vi "JoystickLevel.vi"() -> ()   [LabVIEW 2016]
panel:
  in  "stop":bool
  out "Output":dbl
  in  "MidPower":dbl
  in  "StopThreshold":dbl
  in  "StartThreshold":dbl
  in  "Joystick":dbl(slide) min=-1.0 step=0.01 scale=-1.0..1.0
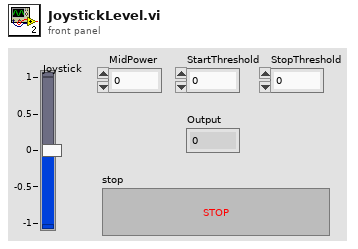
[diagram p1: front panel]
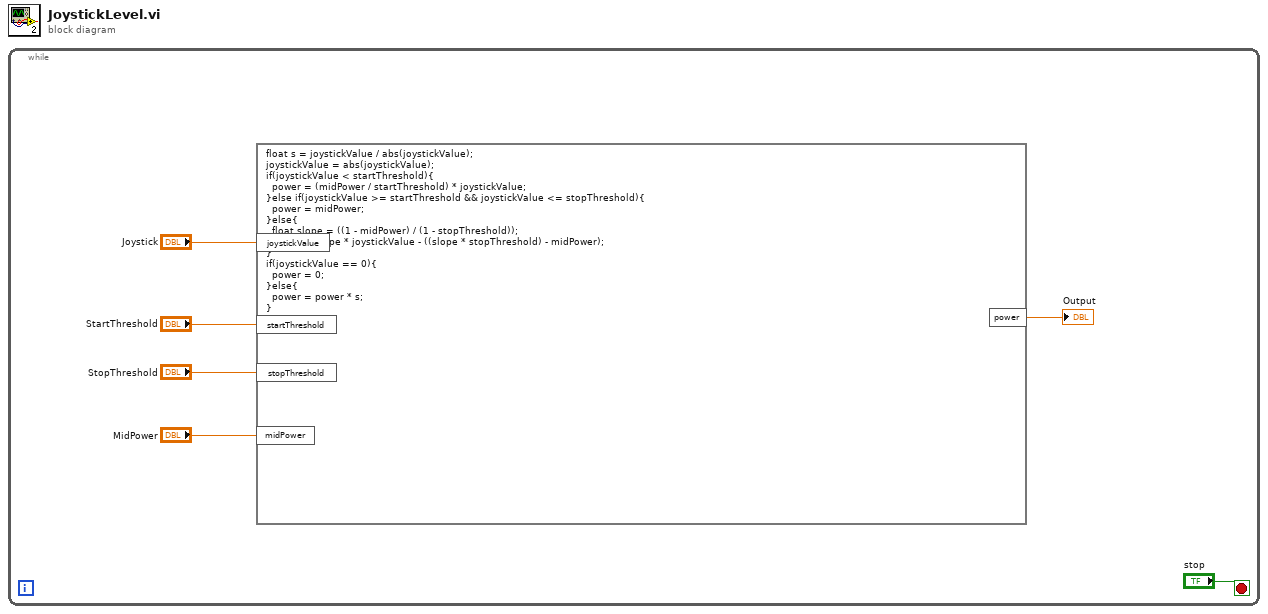
[diagram p0: block diagram]
diagram:
  n1 = while {
    stop <- "stop" stop-if-true
    n2 = formula code="float s = joystickValue / abs(joystickValue);\njoystickValue = abs(joystickValue);\nif(joystickValue < startThreshold){\n  power = (midPower / startThreshold) * joystickValue;\n}else if(joystickValue >= startThreshold && joystickValue <= stopThreshold){\n  power = midPower;\n}else{\n  float slope = ((1 - midPower) / (1 - stopThreshold));\n  power = slope * joystickValue - ((slope * stopThreshold) - midPower);\n}\nif(joystickValue == 0){\n  power = 0;\n}else{\n  power = power * s;\n}"("joystickValue"="Joystick", "startThreshold"="StartThreshold", "stopThreshold"="StopThreshold", "midPower"="MidPower") -> ("power"=→"Output":dbl)
  }
